vi "AO wavefront measure.vi"() -> ()   [LabVIEW 2018]
uses:
  <userlib>/WaveKit.lib/Controls/Image information.ctl
  <userlib>/WaveKit.lib/Controls/Image general information.ctl
  <userlib>/WaveKit.lib/Controls/Image acquisition information.ctl
  <userlib>/WaveKit.lib/Controls/Point2D.ctl
  <userlib>/WaveKit.lib/Controls/Data alignment enum.ctl
  <userlib>/WaveKit.lib/Controls/StatisticsData.ctl
  <userlib>/WaveKit.lib/Classes/Camera/Camera.lvclass
  <userlib>/WaveKit.lib/Classes/CameraSet/CameraSet.lvclass
  <userlib>/WaveKit.lib/Classes/Image/Image.lvclass
  <userlib>/WaveKit.lib/Classes/Phase/Phase.lvclass
  <userlib>/WaveKit.lib/Controls/HasoSlopes.lvclass
  <userlib>/WaveKit.lib/Controls/Pupil.lvclass
panel:
  in  "Filter":u8[](array[numeric])
  out "Phase statistics":T1
  out "Phase values":sgl[][](graph)
  out "Acquisition information":T2={"Image general information"={"Camera serial number"="", "Smearing removed"=FALSE, "Background image removed"=FALSE, "Time Stamp"=timestamp(0 s since 1904-01-01), "Comment"="", "Camera_MAX_Level"=0}, "Acquisition information"={"Exposure duration (us)"=0, "Exposure duration specified (us)"=0, "Gain"=0.0, "Number of summed images"=0, "Trigger type"=""}, "Number of pixels"={"X"=0, "Y"=0}, "Number of bits"=enum."16"}
  in  "Init":bool
  in  "Reset error":bool
  out "exposure_duration_us (get)":u32
  in  "exposure_duration_s (set)":dbl=0.1 min=1.0
  out "Current error":errorcluster
  out "nb_images (get)":u32=10
  in  "nb_images (set)":u32=1 min=1
  in  "Show camera signal":bool
  in  "Exit":bool
  in  "Stop Acq":bool
  in  "Start Acq":bool
  out "Image Camera":u32[][](graph)
  in  "Haso configuration file":path=path "C:/Program Files (x86)/Imagine Optic/Configuration Files/HASO3_first_7364.dat"
  # "Acquisition Parameters"
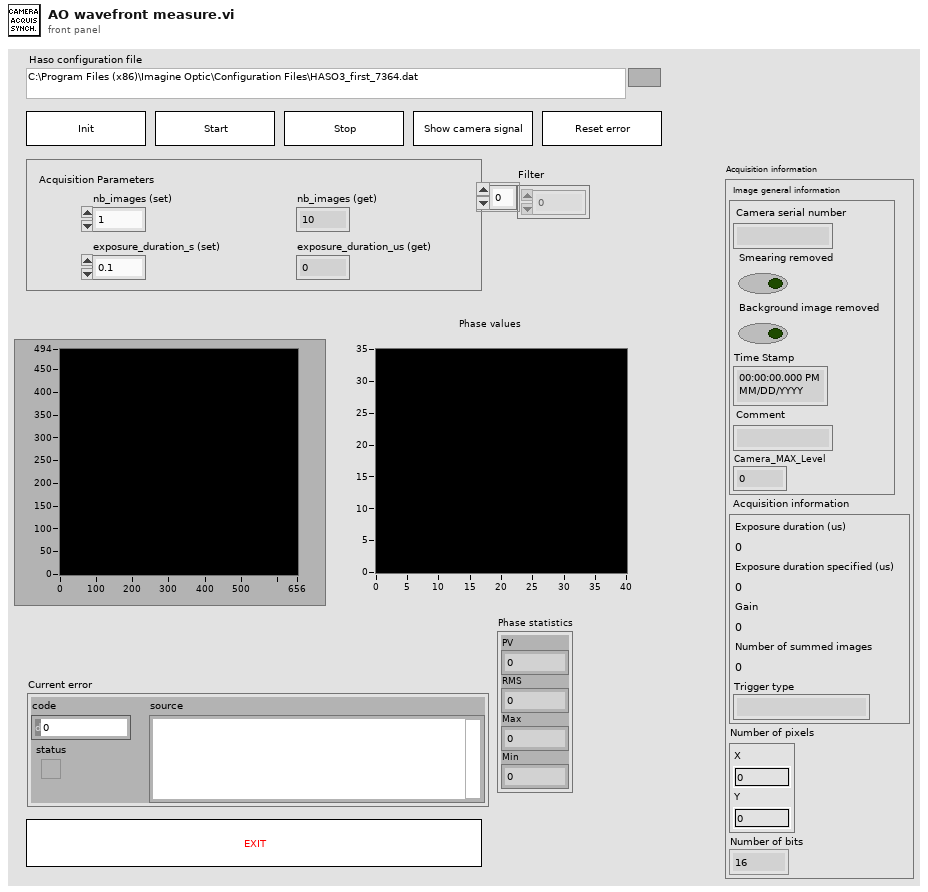
[diagram p1: front panel]
types:
  T1 = typedef "StatisticsData.ctl" = cluster{"PV":sgl, "RMS":dbl, "Max":sgl, "Min":sgl}
  T2 = typedef "Image information.ctl" = cluster{"Image general information":T3, "Acquisition information":T4, "Number of pixels":T5, "Number of bits":T6}
  T3 = typedef "Image general information.ctl" = cluster{"Camera serial number":string, "Smearing removed":bool, "Background image removed":bool, "Time Stamp":timestamp, "Comment":string, "Camera_MAX_Level":i32}
  T4 = typedef "Image acquisition information.ctl" = cluster{"Exposure duration (us)":i32, "Exposure duration specified (us)":i32, "Gain":sgl, "Number of summed images":i32, "Trigger type":string}
  T5 = typedef "Point2D.ctl" = cluster{"X":u32, "Y":u32}
  T6 = typedef "Data alignment enum.ctl" = enum16{"8", "16", "32"}
  T7 = typedef "CameraSpecifications.ctl" = cluster{"Grabber name":string, "Camera name":string, "Camera sn":string, "Pixels_um":T8, "Maximum level":u32, "Data alignment":T6, "Is signed":bool, "Acquisition start":T5, "Acquisition length":T5, "MaxFrameRate_Hz":sgl, "Chip type":enum16{"Progressive scan", "Frame transfert"}}
  T8 = typedef "General dimensions definition.ctl" = cluster{"Size":T5, "Step":T9}
  T9 = typedef "Point2Df.ctl" = cluster{"X":sgl, "Y":sgl}
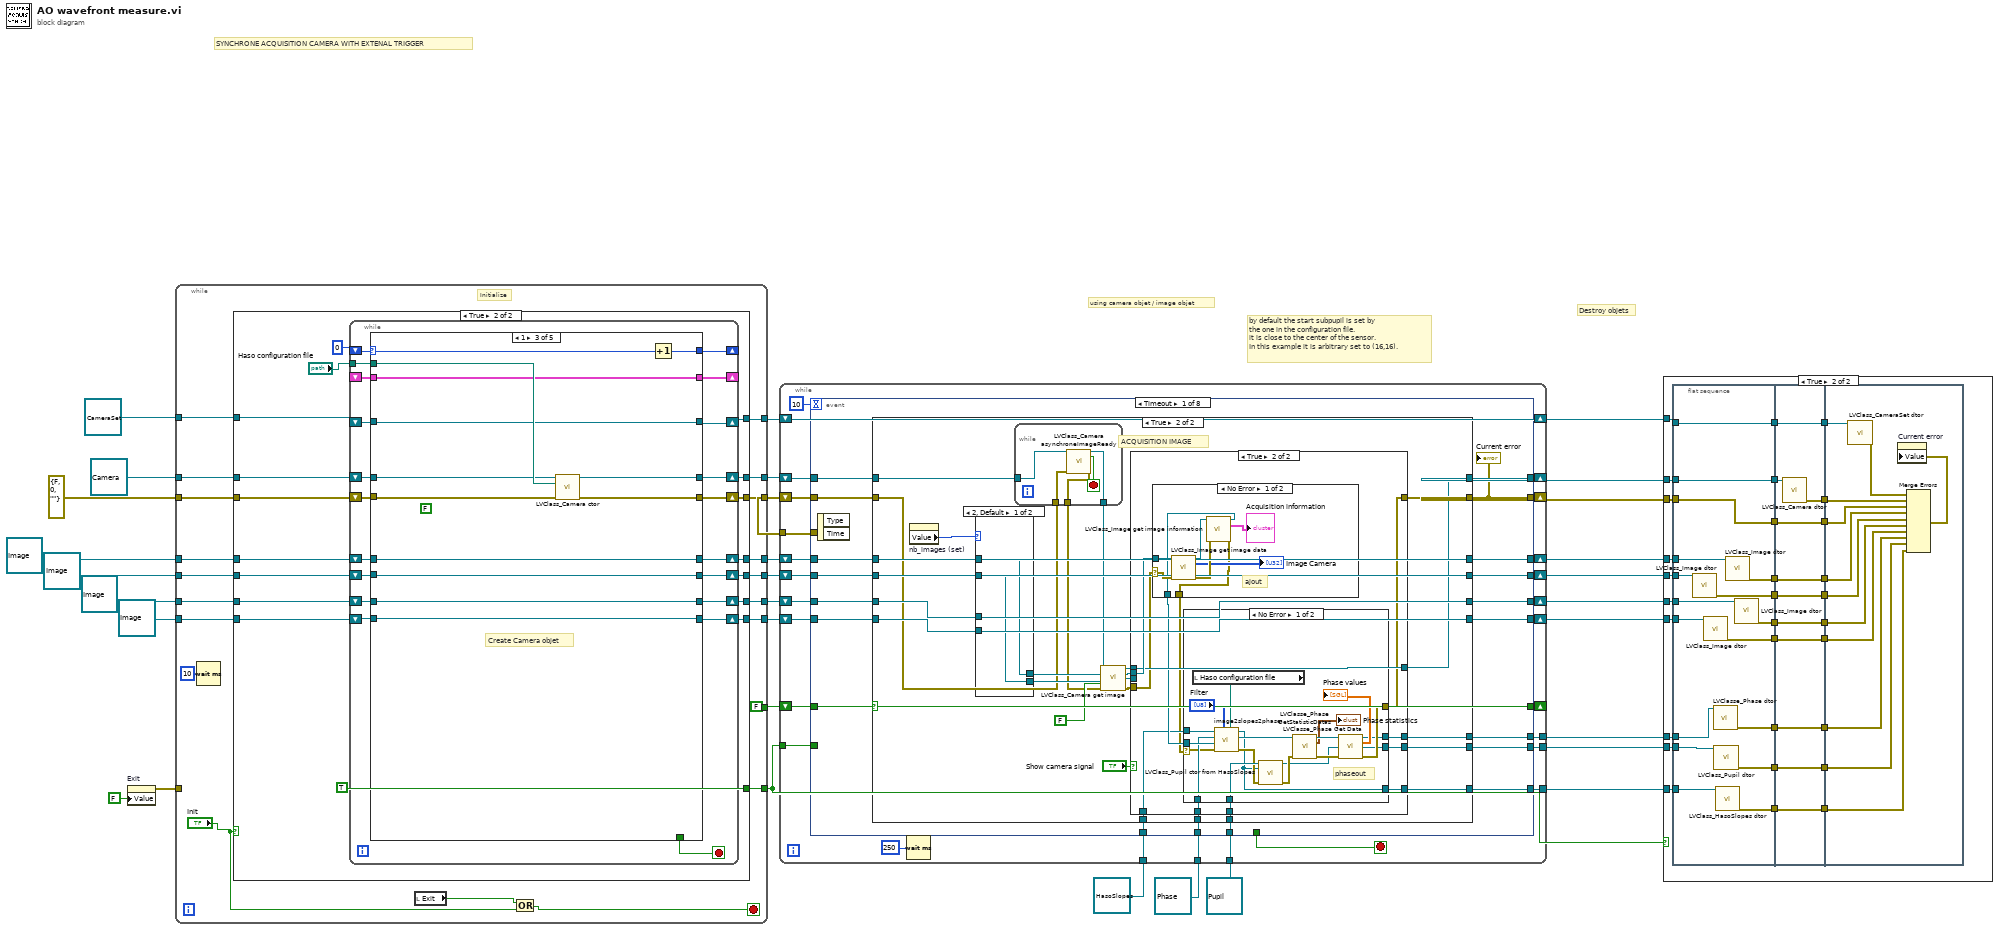
[diagram p0: block diagram]
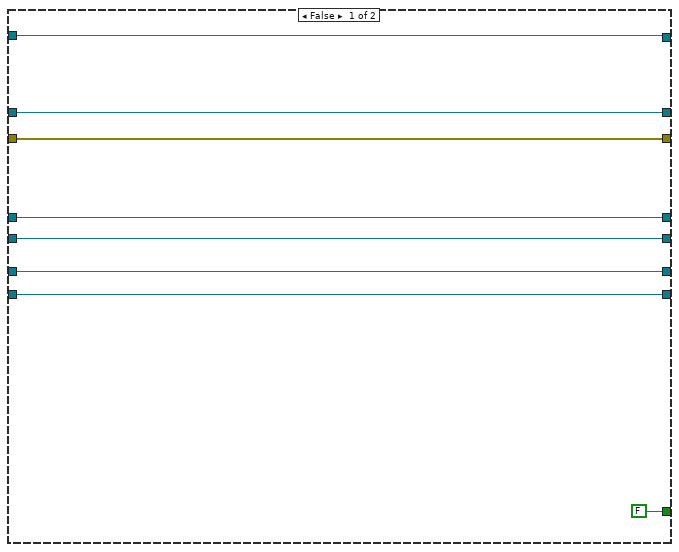
[diagram p3: hidden frame]
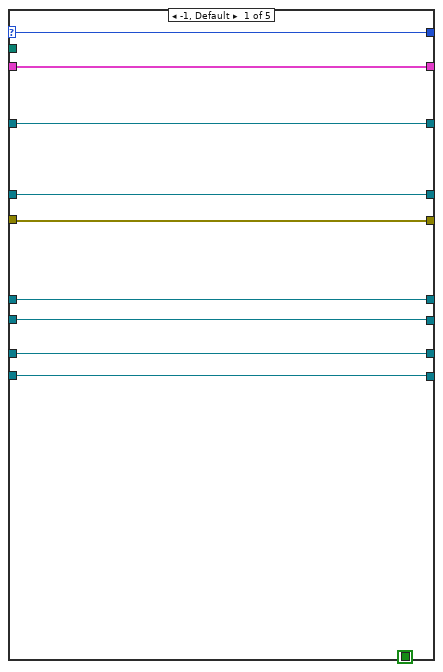
[diagram p4: hidden frame]
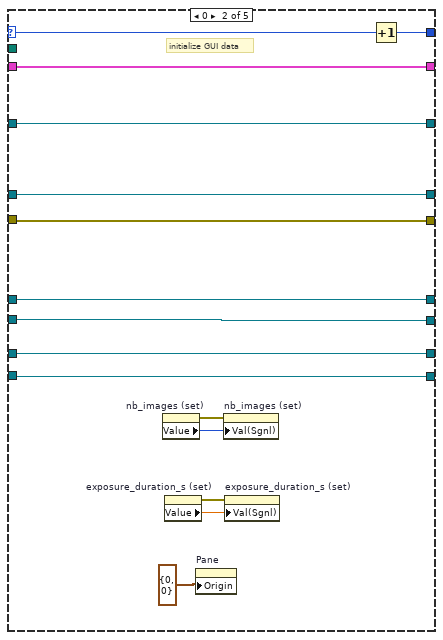
[diagram p5: hidden frame]
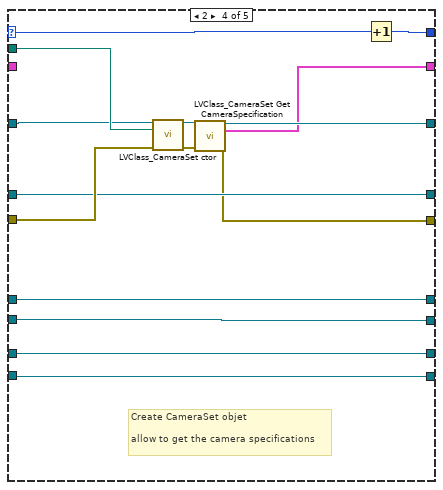
[diagram p6: hidden frame]
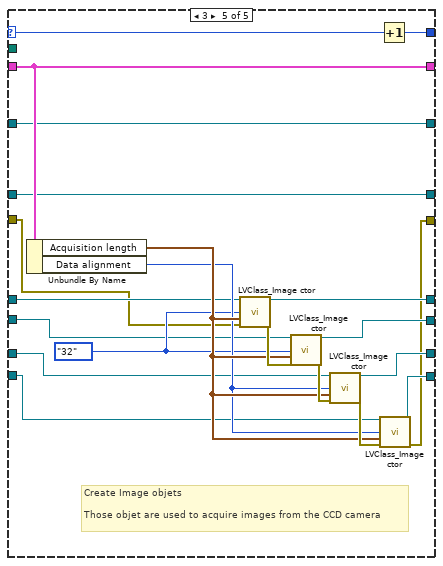
[diagram p7: hidden frame]
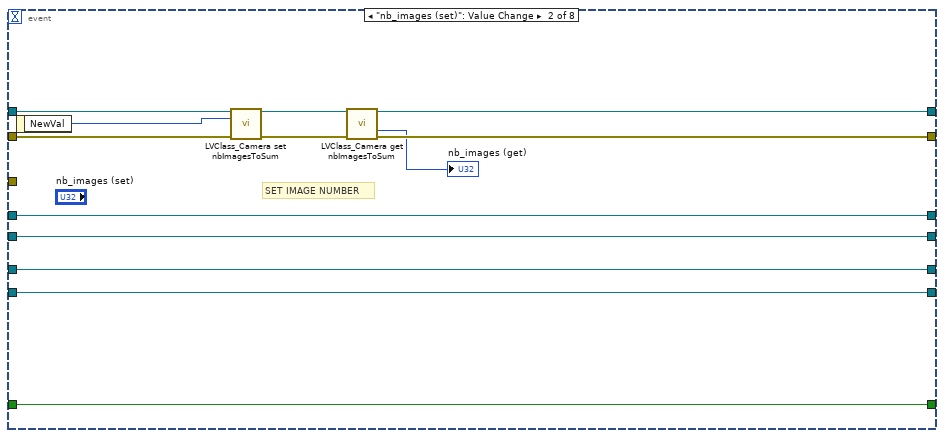
[diagram p13: hidden frame]
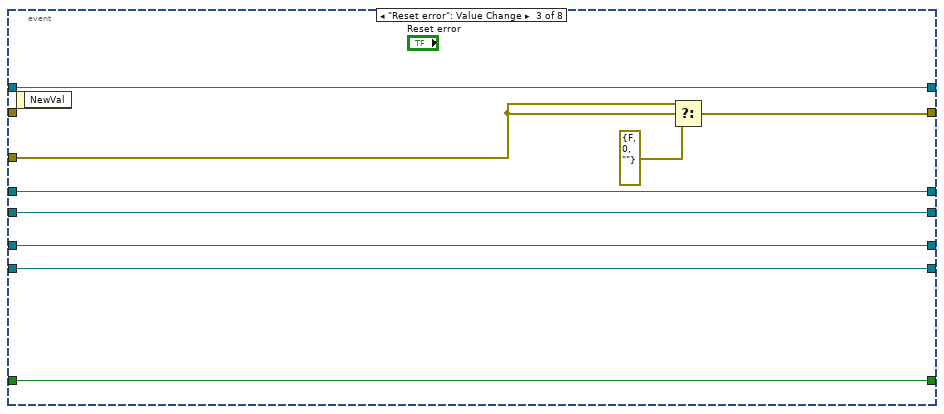
[diagram p14: hidden frame]
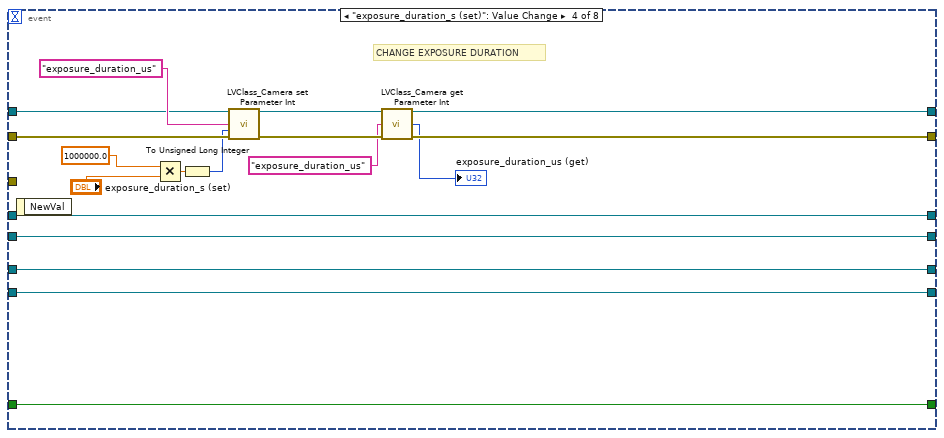
[diagram p15: hidden frame]
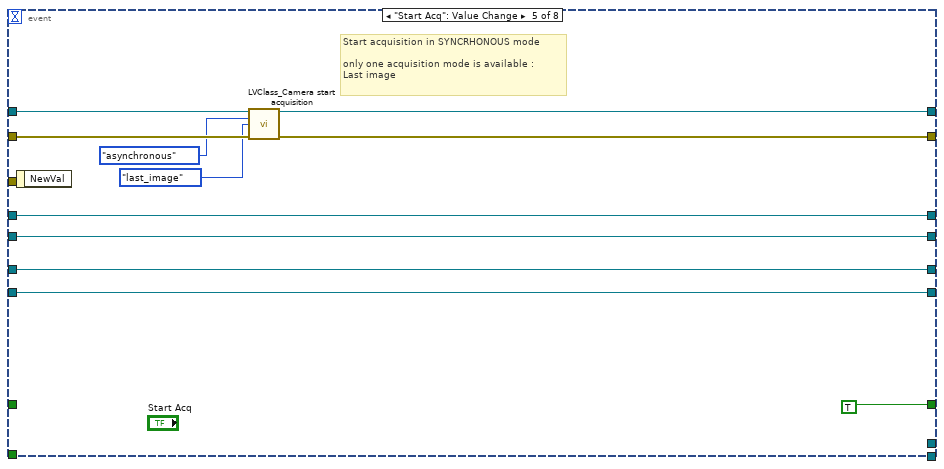
[diagram p16: hidden frame]
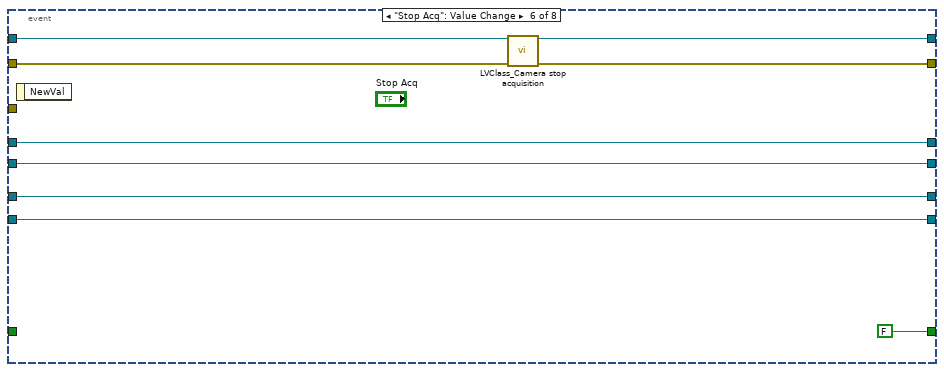
[diagram p17: hidden frame]
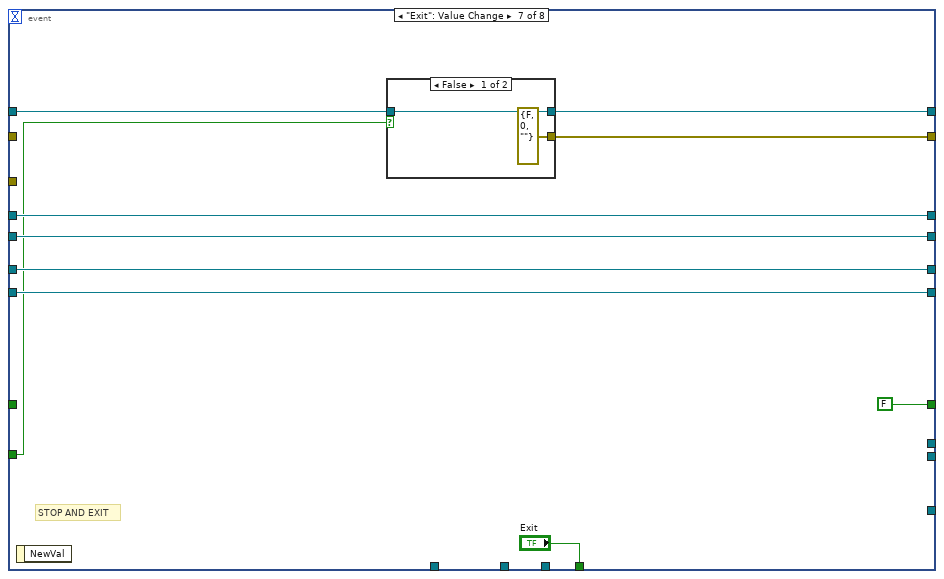
[diagram p18: hidden frame]
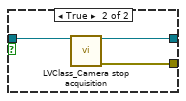
[diagram p19: hidden frame]
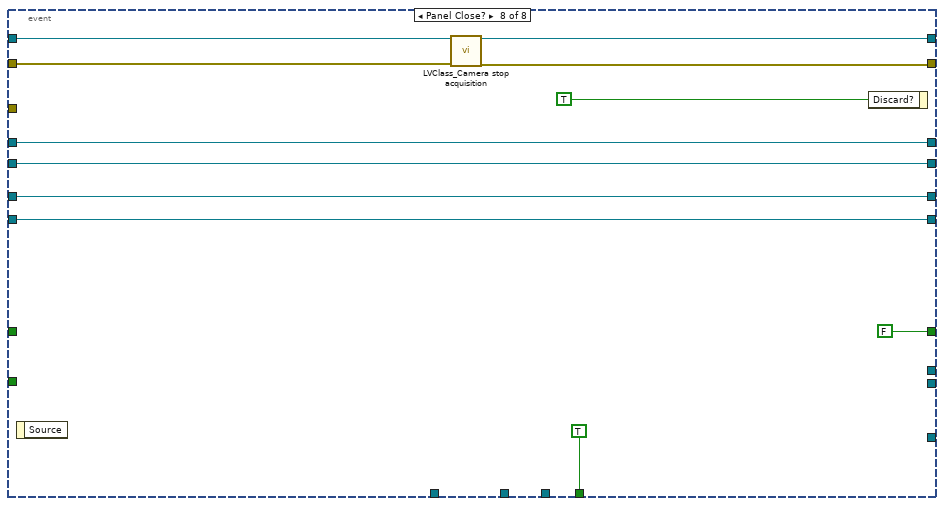
[diagram p20: hidden frame]
diagram:
  # "by default the start subpupil is set by \nthe one in the configuration file. \nit is close to the center of the sensor.\nIn this example it is arbitrary set to (16,16)."
  # "Destroy objets"
  # "using camera objet / image objet"
  # "SYNCHRONE ACQUISITION CAMERA WITH EXTENAL TRIGGER"
  n1 = property on="Exit" class="Bool (strict)"("Value"=FALSE ("Exit")) -> (error out=w7:errorcluster)  [unwired: 2 in, 1 out]
  n2 = while {
    tunnel: [FALSE] -> w24
    tunnel: [w50] -> w23
    tunnel: [w49] -> w22
    tunnel: [w48] -> w21
    tunnel: [w47] -> w20
    tunnel: [w46] -> w19
    tunnel: [w45] -> w18
    tunnel: refnum<class "Camera.lvclass"> refnum ("Camera.lvclass") -> [w44]
    tunnel: refnum<class "CameraSet.lvclass"> refnum ("CameraSet.lvclass") -> [w43]
    tunnel: refnum<class "Image.lvclass"> refnum ("Image in") -> [w42]
    tunnel: refnum<class "Image.lvclass"> refnum ("Image in") -> [w41]
    tunnel: refnum<class "Image.lvclass"> refnum ("Image in") -> [w40]
    tunnel: refnum<class "Image.lvclass"> refnum ("Image in") -> [w39]
    tunnel: errorcluster {"status"=FALSE, "code"=0, "source"=""} ("error out") -> [w38]
    tunnel: [w37] -> w10
    tunnel: [w35] -> w9
    tunnel: w7 -> [_]
    stop <- w32 stop-if-true
    # "Initialize"
    n3 = Wait (ms)(milliseconds to wait=u32 10) -> ()  [unwired: 1 out]
    n4 = case shown="True" "Init" {
      tunnel: [w59 w76] -> w50
      tunnel: [w58 w75] -> w49
      tunnel: [w56 w73] -> w48
      tunnel: [w55 w72] -> w47
      tunnel: [w54 w71] -> w46
      tunnel: [w53 w70] -> w45
      tunnel: w44 -> [w59 w69]
      tunnel: w43 -> [w58 w67]
      tunnel: w42 -> [w56 w66]
      tunnel: w41 -> [w55 w65]
      tunnel: w40 -> [w54 w64]
      tunnel: w39 -> [w53 w63]
      tunnel: w38 -> [w57 w62]
      tunnel: [w57 w61] -> w37
      tunnel: [FALSE TRUE] -> w35
      frame False {
      }
      frame True {
        n5 = while {
          tunnel: "Haso configuration file" -> [w94]
          shift-right: [w96] -> w76
          shift-left: w69 -> [w88]
          shift-right: [w78] -> _
          shift-left: 0 -> [w77]
          shift-right: [w95] -> w75
          shift-left: w67 -> [w87]
          shift-right: [w86] -> _
          shift-left: _ -> [w84]
          shift-right: [w93] -> w73
          shift-left: w66 -> [w85]
          shift-right: [w92] -> w72
          shift-left: w65 -> [w83]
          shift-right: [w91] -> w71
          shift-left: w64 -> [w81]
          shift-right: [w90] -> w70
          shift-left: w63 -> [w82]
          shift-right: [w89] -> w61
          shift-left: w62 -> [w79]
          stop <- w80 stop-if-true
          n6 = case shown="1" w77 {
            tunnel: [w106 w108 w134 w142 w157] -> w96
            tunnel: w94 -> [_ _ w133 w146 _]
            tunnel: [w105 w112 w131 w147 w158] -> w95
            tunnel: [w98 w113 w125 w137 w164] -> w93
            tunnel: [w99 w114 w126 w138 w163] -> w92
            tunnel: [w100 w115 w127 w139 w162] -> w91
            tunnel: [w101 w116 w128 w140 w161] -> w90
            tunnel: [w102 w107 w130 w141 w160] -> w89
            selector: w77 -> [w97 w110 w123 w136 w152]
            tunnel: w88 -> [w106 w108 w132 w142 w157]
            tunnel: w87 -> [w105 w112 w131 w145 w158]
            tunnel: [w103 w109 w129 w144 w159] -> w86
            tunnel: w85 -> [w98 w113 w125 w137 w156]
            tunnel: w84 -> [w103 w109 w129 _ w159]
            tunnel: w83 -> [w99 w114 w126 w138 w155]
            tunnel: w82 -> [w101 w116 w128 w140 w154]
            tunnel: w81 -> [w100 w115 w127 w139 w153]
            tunnel: [TRUE _ _ _ _] -> w80
            tunnel: w79 -> [w102 w107 w122 w143 w150]
            tunnel: [w97 w111 w124 w135 w151] -> w78
            frame -1, Default {
            }
            frame 0 {
              # "initialize GUI data"
              n7 = property on="nb_images (set)" class="DigNum (strict)"() -> (error out=w121:errorcluster, "Value"=w120:u32)  [unwired: 2 in, 1 out]
              n8 = property on="exposure_duration_s (set)" class="DigNum (strict)"() -> (error out=w117:errorcluster, "Value"=w119:dbl)  [unwired: 2 in, 1 out]
              n9 = property on="Pane" class="Pane"("Origin"=cluster{"Horizontal":i16, "Vertical":i16} {"Horizontal"=0, "Vertical"=0} ("Front Panel Window:Origin")) -> ()  [unwired: 2 in, 2 out]
              n10 = property on="nb_images (set)" class="DigNum (strict)"(error in=w121, "Val(Sgnl)"=w120) -> ()  [unwired: 1 in, 2 out]
              n11 = property on="exposure_duration_s (set)" class="DigNum (strict)"(error in=w117, "Val(Sgnl)"=w119) -> ()  [unwired: 1 in, 2 out]
              n12 = Increment(x=w110) -> (x+1=w111:i32)
            }
            frame 1 {
              (unwired) FALSE ("Acq required")
              # "Create Camera objet"
              n13 = call <userlib>:"LVClass_Camera ctor.vi"("Camera"=w132, "Configuration file path"=w133, "error in (no error)"=w122) -> ("Camera (new)"=w134:refnum<class "Camera.lvclass">, "error out"=w130:errorcluster)  [unwired: 11 in]
              n14 = Increment(x=w123) -> (x+1=w124:i32)
            }
            frame 2 {
              # "Create CameraSet objet\n\nallow to get the camera specifications"
              n15 = call <userlib>:"LVClass_CameraSet ctor.vi"("CameraSet.lvclass"=w145, "Configuration file path"=w146, "error in (no error)"=w143) -> ("CameraSet.lvclass"=w149:refnum<class "CameraSet.lvclass">, "error out"=w148:errorcluster)  [unwired: 11 in]
              n16 = call <userlib>:"LVClass_CameraSet Get CameraSpecification.vi"("CameraSet.lvclass"=w149, "error in (no error)"=w148) -> ("CameraSet.lvclass"=w147:refnum<class "CameraSet.lvclass">, "Camera Config"=w144:T7, "error out"=w141:errorcluster)  [unwired: 11 in]
              n17 = Increment(x=w136) -> (x+1=w135:i32)
            }
            frame 3 {
              w165 = Data_alignment_enum."32" ("Data alignment")
              # "Create Image objets\n\nThose objet are used to acquire images from the CCD camera"
              n18 = Unbundle By Name(w159) -> ("Acquisition length"=w167:T5, "Data alignment"=w166:T6)
              n19 = call <userlib>:"LVClass_Image ctor.vi"("Image in"=w156, "Data alignment"=w165, "Size"=w167, "error in (no error)"=w150) -> ("Image out"=w164:refnum<class "Image.lvclass">, "error out"=w168:errorcluster)  [unwired: 10 in]
              n20 = call <userlib>:"LVClass_Image ctor.vi"("Image in"=w155, "Data alignment"=w165, "Size"=w167, "error in (no error)"=w168) -> ("Image out"=w163:refnum<class "Image.lvclass">, "error out"=w169:errorcluster)  [unwired: 10 in]
              n21 = call <userlib>:"LVClass_Image ctor.vi"("Image in"=w153, "Data alignment"=w166, "Size"=w167, "error in (no error)"=w169) -> ("Image out"=w162:refnum<class "Image.lvclass">, "error out"=w170:errorcluster)  [unwired: 10 in]
              n22 = Increment(x=w152) -> (x+1=w151:i32)
              n23 = call <userlib>:"LVClass_Image ctor.vi"("Image in"=w154, "Data alignment"=w166, "Size"=w167, "error in (no error)"=w170) -> ("Image out"=w161:refnum<class "Image.lvclass">, "error out"=w160:errorcluster)  [unwired: 10 in]
            }
          }
        }
      }
    }
    n24 = local read "Exit"() -> (w34:bool)
    n25 = Or(x=w34, y="Init") -> (x .or. y?=w32:bool)
  }
  n26 = while {
    shift-right: [w193] -> w31
    shift-left: w10 -> [w195]
    shift-right: [w191] -> w30
    shift-left: w23 -> [w192]
    shift-right: [w185] -> w29
    shift-left: w21 -> [w190]
    shift-right: [w184] -> w28
    shift-left: w20 -> [w189]
    shift-right: [w183] -> w27
    shift-left: w19 -> [w188]
    shift-right: [w182] -> w26
    shift-left: w18 -> [w187]
    shift-right: [w181] -> _
    shift-left: w24 -> [w186]
    shift-right: [w180] -> w25
    shift-left: w22 -> [w180]
    tunnel: w10 -> [w179]
    tunnel: w9 -> [w178]
    tunnel: refnum<class "Phase.lvclass"> refnum ("Phase in") -> [w177]
    tunnel: [w176] -> w5
    tunnel: [w175] -> w4
    tunnel: refnum<class "HasoSlopes.lvclass"> refnum ("HasoSlopes in") -> [w173]
    tunnel: refnum<class "Pupil.lvclass"> refnum ("Pupil in") -> [w172]
    tunnel: [w171] -> w1
    stop <- w194 stop-if-true
    n27 = event shown="[0] Timeout" {
      selector: _ -> [_ _ _ _ _ _ _ _]
      dyn-events: _ -> [_ _ _ _ _ _ _ _]
      timeout: 10 -> [_ _ _ _ _ _ _ _]
      tunnel: w195 -> [w207 w320 _ w347 w358 w360 _ w385]
      tunnel: [_ _ _ _ _ _ "Exit" TRUE ("Exit")] -> w194
      tunnel: [w203 w318 w323 w342 w356 w366 w376 w390] -> w193
      tunnel: w192 -> [w212 w319 w325 w346 w359 w367 w377 w392]
      tunnel: [w211 w317 w325 w343 w357 w368 w375 w391] -> w191
      tunnel: w190 -> [w215 w310 w327 w336 w353 w362 w371 w386]
      tunnel: w189 -> [w214 w311 w328 w337 w352 w363 w372 w387]
      tunnel: w188 -> [w213 w312 w329 w338 w351 w364 w373 w388]
      tunnel: w187 -> [w208 w313 w330 w339 w350 w365 w374 w389]
      tunnel: w186 -> [w204 w309 w326 w335 _ _ _ _]
      tunnel: [w210 w310 w327 w336 w353 w362 w371 w386] -> w185
      tunnel: [w209 w311 w328 w337 w352 w363 w372 w387] -> w184
      tunnel: [w206 w312 w329 w338 w351 w364 w373 w388] -> w183
      tunnel: [w205 w313 w330 w339 w350 w365 w374 w389] -> w182
      tunnel: [w204 w309 w326 w335 TRUE FALSE FALSE FALSE] -> w181
      tunnel: w179 -> [_ _ w322 _ _ _ _ _]
      tunnel: w178 -> [_ _ _ _ _ _ w369 _]
      tunnel: w177 -> [w202 _ _ _ _ _ _ _]
      tunnel: [w201 _ _ _ _ _ _ _] -> w176
      tunnel: [w200 _ _ _ _ _ _ _] -> w175
      tunnel: w173 -> [w199 _ _ _ _ _ _ _]
      tunnel: w172 -> [w198 _ _ _ _ _ _ _]
      tunnel: [w197 _ _ _ _ _ _ _] -> w171
      event Timeout {
        n28 = event-data() -> ()  [unwired: 1 in, 2 out]
        n29 = case shown="True" w204 {
          tunnel: [w219 w239] -> w203
          tunnel: w215 -> [w224 w245]
          tunnel: [w224 w245] -> w210
          tunnel: [w220 w236] -> w209
          tunnel: w213 -> [w223 w244]
          tunnel: w208 -> [w222 w243]
          tunnel: [w223 w244] -> w206
          tunnel: [w222 w243] -> w205
          tunnel: w214 -> [w220 w236]
          tunnel: w212 -> [w221 w234]
          tunnel: [w221 w235] -> w211
          tunnel: w207 -> [w219 w232]
          tunnel: w202 -> [w218 w230]
          tunnel: [w217 w229] -> w201
          tunnel: [w218 w228] -> w200
          tunnel: w199 -> [w216 w227]
          tunnel: w198 -> [w217 w226]
          tunnel: [w216 w225] -> w197
          frame False {
          }
          frame True {
            # "ACQUISITION IMAGE"
            n30 = property on="nb_images (set)" class="DigNum (strict)"() -> ("Value"=w246:u32)  [unwired: 2 in, 2 out]
            n31 = case shown="2, Default" w246 {
              tunnel: [w256 w258] -> w247
              tunnel: w236 -> [w255 _]
              tunnel: w245 -> [w256 _]
              tunnel: [w255 w257] -> w242
              tunnel: w244 -> [_ w258]
              tunnel: w243 -> [_ w257]
              frame 2, Default {
              }
              frame 1 {
              }
            }
            n32 = while {
              tunnel: w234 -> [w254]
              tunnel: [w253] -> w233
              tunnel: w232 -> [w251]
              tunnel: [w250] -> w231
              stop <- w252 stop-if-true
              n33 = call <userlib>:"LVClass_Camera asynchroneImageReady.vi"("Camera in"=w254, "error in (no error)"=w251) -> ("Camera out"=w253:refnum<class "Camera.lvclass">, "ready"=w252:bool, "error out"=w250:errorcluster)  [unwired: 11 in]
            }
            n34 = call <userlib>:"LVClass_Camera get image.vi"("Camera in"=w233, "Image"=w247, "Image RAW"=w242, "remove_background"=FALSE, "error in (no error)"=w231) -> ("Camera out"=w249:refnum<class "Camera.lvclass">, "Image (dup)"=w240:refnum<class "Image.lvclass">, "Image (dup) RAW"=w241:refnum<class "Image.lvclass">, "error out"=w237:errorcluster)  [unwired: 7 in]
            n35 = case shown="True" "Show camera signal" {
              tunnel: w249 -> [w263 w274]
              tunnel: w240 -> [_ w275]
              tunnel: w237 -> [w262 w273]
              tunnel: [w263 w274] -> w235
              tunnel: [w262 w271] -> w239
              tunnel: w241 -> [_ _]
              tunnel: w230 -> [w261 w270]
              tunnel: [w260 w269] -> w229
              tunnel: [w261 w268] -> w228
              tunnel: w227 -> [w259 w267]
              tunnel: w226 -> [w260 w265]
              tunnel: [w259 w264] -> w225
              frame False {
              }
              frame True {
                n36 = case shown="No Error" w273 {
                  selector: w273 -> [w306 w307]
                  tunnel: w275 -> [w303 w308]
                  tunnel: [w300 w308] -> w272
                  tunnel: [w299 w307] -> w266
                  frame No Error {
                    # "ajout"
                    n37 = call <userlib>:"LVClass_Image get image data.vi"("Image in"=w303, "error in (no error)"=w306) -> ("Image out"=w305:refnum<class "Image.lvclass">, "Image data out"=→"Image Camera":u32[][], "error out"=w304:errorcluster)  [unwired: 11 in]
                    n38 = call <userlib>:"LVClass_Image get image information.vi"("Image in"=w305, "error in (no error)"=w304) -> ("Image out"=w300:refnum<class "Image.lvclass">, "Acquisition information"=→"Acquisition information":T2, "error out"=w299:errorcluster)  [unwired: 11 in]
                  }
                  frame Error {
                  }
                }
                n39 = case shown="No Error" w266 {
                  selector: w266 -> [w281 w298]
                  tunnel: [w292 w298] -> w271
                  tunnel: w272 -> [w284 _]
                  tunnel: w270 -> [w283 w297]
                  tunnel: [w289 w296] -> w269
                  tunnel: [w288 w297] -> w268
                  tunnel: w267 -> [w282 w295]
                  tunnel: w265 -> [w280 w296]
                  tunnel: [w276 w295] -> w264
                  frame No Error {
                    # "phaseout"
                    n40 = local read "Haso configuration file"() -> (w287:path)
                    n41 = call "image2slopes2phase.vi"("Haso configuration file"=w287, "Filter"="Filter", "error in (no error)"=w281, "Image in"=w284, "Phase in"=w283, "HasoSlopes in"=w282) -> ("error out"=w279:errorcluster, "Phase out"=w285:refnum<class "Phase.lvclass">, "HasoSlopes out"=w276:refnum<class "HasoSlopes.lvclass">)  [unwired: 2 in, 1 out]
                    n42 = call <userlib>:"LVClass_Pupil ctor from HasoSlopes.vi"("Pupil in"=w280, "HasoSlopes.lvclass"=w276, "error in (no error)"=w279) -> ("Pupil out"=w277:refnum<class "Pupil.lvclass">, "error out"=w278:errorcluster)  [unwired: 11 in]
                    n43 = call <userlib>:"LVClasse_Phase GetStatisticDatas.vi"("Phase in"=w285, "error in (no error)"=w278) -> ("Phase out"=w294:refnum<class "Phase.lvclass">, "StatisticsData"=→"Phase statistics":T1, "error out"=w290:errorcluster)  [unwired: 11 in]
                    n44 = call <userlib>:"LVClasse_Phase Get Data.vi"("Phase in"=w294, "Pupil"=w277, "error in (no error)"=w290) -> ("Phase out"=w288:refnum<class "Phase.lvclass">, "data"=→"Phase values":sgl[][], "Pupil (dup)"=w289:refnum<class "Pupil.lvclass">, "error out"=w292:errorcluster)  [unwired: 9 in]
                  }
                  frame Error {
                  }
                }
              }
            }
          }
        }
        "Current error" <- w203
      }
      event "nb_images (set)": Value Change {
        # "SET IMAGE NUMBER"
        n45 = event-data() -> ("NewVal"=w321:u32)  [unwired: 1 in]
        n46 = call <userlib>:"LVClass_Camera set nbImagesToSum.vi"("Camera in"=w319, "nb_image"=w321, "error in (no error)"=w320) -> ("Camera out"=w316:refnum<class "Camera.lvclass">, "error out"=w315:errorcluster)  [unwired: 11 in]
        n47 = call <userlib>:"LVClass_Camera get nbImagesToSum.vi"("Camera in"=w316, "error in (no error)"=w315) -> ("Camera out"=w317:refnum<class "Camera.lvclass">, "nb_image"=→"nb_images (get)":u32, "error out"=w318:errorcluster)  [unwired: 11 in]
      }
      event "Reset error": Value Change {
        n48 = event-data() -> ()  [unwired: 1 in, 1 out]
        n49 = Select(t=w322, s=w322, f=errorcluster {"status"=FALSE, "code"=0, "source"=""} ("error out")) -> (s? t:f=w323:errorcluster)
      }
      event "exposure_duration_s (set)": Value Change {
        # "CHANGE EXPOSURE DURATION"
        n50 = event-data() -> ()  [unwired: 1 in, 1 out]
        n51 = Multiply(x=1000000.0, y="exposure_duration_s (set)") -> (x*y=w333:dbl)
        n52 = To Unsigned Long Integer(number=w333) -> (unsigned 32bit integer=w332:u32)
        n53 = call <userlib>:"LVClass_Camera set Parameter Int.vi"("Camera in"=w346, "parameter_name"="exposure_duration_us", "value"=w332, "error in (no error)"=w347) -> ("Camera out"=w345:refnum<class "Camera.lvclass">, "error out"=w344:errorcluster)  [unwired: 10 in]
        n54 = call <userlib>:"LVClass_Camera get Parameter Int.vi"("Camera in"=w345, "parameter_name"="exposure_duration_us", "error in (no error)"=w344) -> ("Camera out"=w343:refnum<class "Camera.lvclass">, "value"=→"exposure_duration_us (get)":i32, "error out"=w342:errorcluster)  [unwired: 10 in]
      }
      event "Start Acq": Value Change {
        # "Start acquisition in SYNCRHONOUS mode\n\nonly one acquisition mode is available :\nLast image"
        n55 = event-data() -> ()  [unwired: 1 in, 1 out]
        n56 = call <userlib>:"LVClass_Camera start acquisition.vi"("Camera in"=w359, "synchronisation_mode"=enum16{"synchronous", "asynchronous"}."asynchronous", "acquisition_mode"=enum16{"last_image", "new_image"}."last_image", "error in (no error)"=w358) -> ("Camera out"=w357:refnum<class "Camera.lvclass">, "error out"=w356:errorcluster)  [unwired: 10 in]
      }
      event "Stop Acq": Value Change {
        n57 = event-data() -> ()  [unwired: 1 in, 1 out]
        n58 = call <userlib>:"LVClass_Camera stop acquisition.vi"("Camera in"=w367, "error in (no error)"=w360) -> ("Camera out"=w368:refnum<class "Camera.lvclass">, "error out"=w366:errorcluster)  [unwired: 12 in]
      }
      event "Exit": Value Change {
        # "STOP AND EXIT"
        n59 = event-data() -> ()  [unwired: 1 in, 1 out]
        n60 = case shown="False" w369 {
          tunnel: w377 -> [w380 w383]
          tunnel: [errorcluster {"status"=FALSE, "code"=0, "source"=""} ("error out") w382] -> w376
          tunnel: [w380 w381] -> w375
          frame False {
          }
          frame True {
            n61 = call <userlib>:"LVClass_Camera stop acquisition.vi"("Camera in"=w383) -> ("Camera out"=w381:refnum<class "Camera.lvclass">, "error out"=w382:errorcluster)  [unwired: 13 in]
          }
        }
      }
      event Panel Close? {
        n62 = event-data() -> ()  [unwired: 1 in, 1 out]
        n63 = call <userlib>:"LVClass_Camera stop acquisition.vi"("Camera in"=w392, "error in (no error)"=w385) -> ("Camera out"=w391:refnum<class "Camera.lvclass">, "error out"=w390:errorcluster)  [unwired: 12 in]
        n64 = event-data("Discard?"=TRUE) -> ()  [unwired: 1 in, 1 out]
      }
    }
    n65 = Wait (ms)(milliseconds to wait=u32 250) -> ()  [unwired: 1 out]
  }
  n66 = case shown="True" w9 {
    tunnel: w31 -> [_ w410]
    tunnel: w30 -> [_ w409]
    tunnel: w29 -> [_ w408]
    tunnel: w28 -> [_ w407]
    tunnel: w27 -> [_ w406]
    tunnel: w26 -> [_ w405]
    tunnel: w25 -> [_ w404]
    tunnel: w5 -> [_ w403]
    tunnel: w4 -> [_ w402]
    tunnel: w1 -> [_ w395]
    frame False {
    }
    frame True {
      n67 = flat-sequence {
        tunnel: w409 -> [w441]
        tunnel: w410 -> [w439]
        tunnel: [w441] -> w424
        tunnel: w404 -> [w440]
        tunnel: [w440] -> w423
        tunnel: [w439] -> w422
        tunnel: w408 -> [w438]
        tunnel: w407 -> [w437]
        tunnel: w406 -> [w436]
        tunnel: w405 -> [w435]
        tunnel: [w434] -> w421
        tunnel: [w433] -> w420
        tunnel: [w432] -> w419
        tunnel: [w431] -> w418
        tunnel: w403 -> [w430]
        tunnel: w402 -> [w429]
        tunnel: [w426] -> w400
        tunnel: [w428] -> w398
        tunnel: [w427] -> w396
        tunnel: w395 -> [w425]
        tunnel: w424 -> [w452]
        tunnel: w423 -> [w451]
        tunnel: w422 -> [w449]
        tunnel: [w451] -> w417
        tunnel: [w450] -> w416
        tunnel: [w449] -> w415
        tunnel: w421 -> [w448]
        tunnel: [w448] -> w414
        tunnel: w420 -> [w447]
        tunnel: [w447] -> w413
        tunnel: w419 -> [w446]
        tunnel: [w446] -> w412
        tunnel: w418 -> [w445]
        tunnel: [w445] -> w411
        tunnel: [w444] -> w401
        tunnel: w400 -> [w444]
        tunnel: [w443] -> w399
        tunnel: w398 -> [w443]
        tunnel: [w442] -> w397
        tunnel: w396 -> [w442]
        tunnel: w417 -> [w464]
        tunnel: w416 -> [w462]
        tunnel: w415 -> [w461]
        tunnel: w414 -> [w460]
        tunnel: w413 -> [w459]
        tunnel: w412 -> [w458]
        tunnel: w411 -> [w457]
        tunnel: w401 -> [w455]
        tunnel: w399 -> [w454]
        tunnel: w397 -> [w453]
        frame #0 {
          n68 = call <userlib>:"LVClass_Image dtor.vi"("Image in"=w437) -> ("error out"=w433:errorcluster)  [unwired: 13 in, 1 out]
          n69 = call <userlib>:"LVClass_Image dtor.vi"("Image in"=w435) -> ("error out"=w431:errorcluster)  [unwired: 13 in, 1 out]
          n70 = call <userlib>:"LVClasse_Phase dtor.vi"("Phase in"=w429) -> ("error out"=w427:errorcluster)  [unwired: 13 in, 1 out]
          n71 = call <userlib>:"LVClass_Pupil dtor.vi"("Pupil in"=w430) -> ("error out"=w428:errorcluster)  [unwired: 13 in, 1 out]
          n72 = call <userlib>:"LVClass_HasoSlopes dtor.vi"("HasoSlopes in"=w425) -> ("error out"=w426:errorcluster)  [unwired: 13 in, 1 out]
          n73 = call <userlib>:"LVClass_Image dtor.vi"("Image in"=w438) -> ("error out"=w434:errorcluster)  [unwired: 13 in, 1 out]
          n74 = call <userlib>:"LVClass_Image dtor.vi"("Image in"=w436) -> ("error out"=w432:errorcluster)  [unwired: 13 in, 1 out]
        }
        frame #1 {
          n75 = call <userlib>:"LVClass_Camera dtor.vi"("Camera in"=w452) -> ("error out"=w450:errorcluster)  [unwired: 13 in, 1 out]
        }
        frame #2 {
          n76 = call <userlib>:"LVClass_CameraSet dtor.vi"("CameraSet.lvclass"=w464) -> ("error out"=w463:errorcluster)  [unwired: 13 in, 1 out]
          n77 = Merge Errors(w463, w462, w461, w460, w459, w458, w457, w453, w454, w455) -> (w456:errorcluster)
          n78 = property on="Current error" class="Clust (strict)"("Value"=w456) -> ()  [unwired: 2 in, 2 out]
        }
      }
    }
  }
